vi "Constants.vi"() -> ()   [LabVIEW 2015, in "AIT 429 Shared.lvlib"]
doc: "Use this Global VI to access the GUIDs assigned to the page resources of the Custom Device."
uses:
  AIT 429 Shared.lvlib
panel:
  in  "Tab Control":enum32{"GUIDS", "Constants", "Properties"}(tab)
  in  "Status Section Page":string="d47aa00e-f699-4d59-94c0-e2f1966f44aa"
  in  "AIT 429 Word Page":string="c976e646-a24d-488b-9d95-5bd8d1727224"
  in  "AIT 429 Parameter Page":string="e9f79bde-5caf-4b2b-afe3-0ce1e606e7c7"
  in  "AIT 429 Outputs Page":string="3512d02a-2029-43cc-b95c-a92ed63679f7"
  in  "AIT 429 Label Page":string="d344d039-fb12-41b4-81fc-ed75cdddcb8d"
  in  "AIT 429 Inputs Page":string="6b205014-7e01-4dc7-9fb4-ec708a1264b1"
  in  "AIT 429 ARINC Channel Page":string="2ea04988-eee4-4e83-9dd8-12eaea61e539"
  in  "AIT 429 Custom Device":string="6de686c8-271d-4eac-aefc-5952b5c6028a"
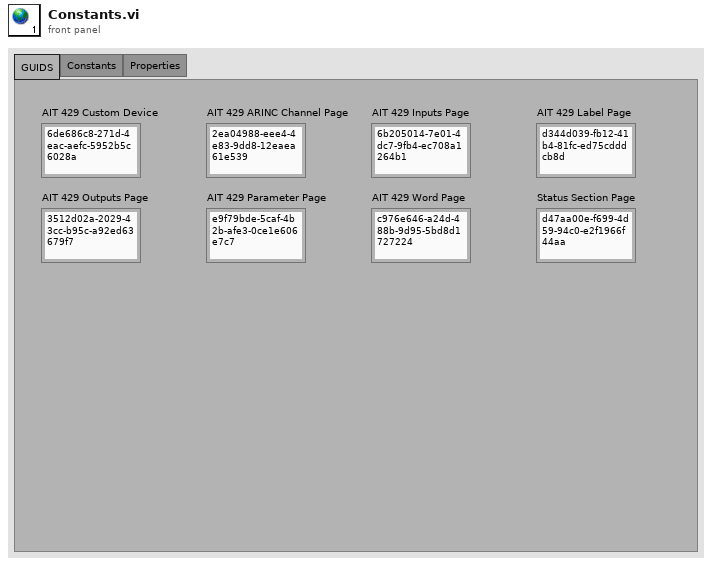
[diagram p1: front panel]
diagram:
